vi "Wait for Logger Init.vi"(8 "error in (no error)":errorcluster, 10 "Timeout (ms)":u32=1000) -> (0 "error out":errorcluster)   [LabVIEW 2016, in "hse-logger.lvlib"]
doc: "Check if the Logger is initilized and waits until it is initilized or a timeout occurs.\n\nWire <b>-1</b> to Timeout to wait a undefined time.\n\nDefault Timeout is 1000 ms.\n\n____\n(c) HAMPEL SOFTWARE ENGINEERING"
uses:
  hse-logger.lvlib
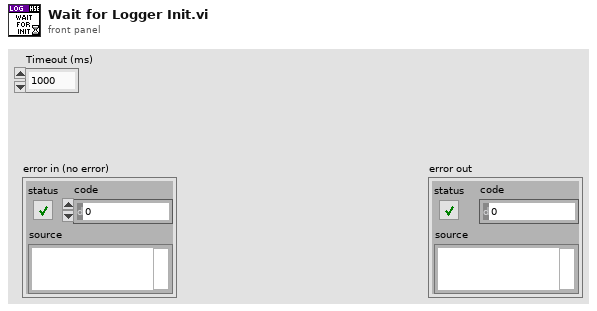
[diagram p1: front panel]
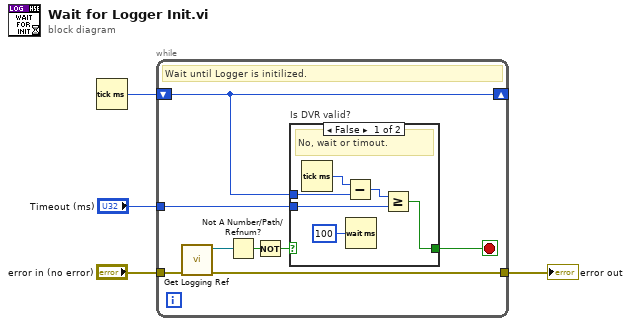
[diagram p0: block diagram]
diagram:
  n1 = Tick Count (ms)() -> (millisecond timer value=w2:u32)
  n2 = while {
    tunnel: "error in (no error)" -> [w12]
    tunnel: [w10] -> w4
    shift-right: [w6] -> _
    shift-left: w2 -> [w6]
    tunnel: "Timeout (ms)" -> [w5]
    stop <- w7 stop-if-true
    # "Wait until Logger is initilized."
    n3 = call "Get Logging Ref.vi"("error in"=w12) -> ("error out"=w10:errorcluster, "Logger DVR"=w11:refnum<data-value>)  [unwired: 9 in]
    n4 = Not A Number/Path/Refnum?(number/path/refnum=w11) -> (NaN/Path/Refnum?=w9:bool)
    n5 = Not(x=w9) -> (.not. x?=w8:bool)
    n6 = case "Is DVR valid?" shown="False" w8 {
      selector: w8 -> [_ w19]
      tunnel: [w14 w19] -> w7
      tunnel: w6 -> [w17 _]
      tunnel: w5 -> [w15 _]
      frame False {
        # "No, wait or timout."
        n7 = Tick Count (ms)() -> (millisecond timer value=w18:u32)
        n8 = Subtract(x=w18, y=w17) -> (x-y=w16:u32)
        n9 = Wait (ms)(milliseconds to wait=u32 100) -> ()  [unwired: 1 out]
        n10 = Greater Or Equal?(x=w16, y=w15) -> (x >= y?=w14:bool)
      }
      frame True {
        # "Yes"
      }
    }
  }
  "error out" <- w4
